vi "VCS Set Quick Stop State.vi"(8 "error in (no error)":errorcluster, 11 "axis in":cluster{"keyHandle":u32, "nodeId":u16}={"keyHandle"=0, "nodeId"=1}) -> (0 "error out":errorcluster, 3 "axis out":cluster{"keyHandle":u32, "nodeId":u16}={"keyHandle"=0, "nodeId"=1})   [LabVIEW 2019]
doc: "<B>VCS Set Quick Stop State</B> the device changes to quick stop state."
uses:
  Resources/EposCmd.dll
  Resources/EposCmd64.dll
panel:
  in  "pErrorCode":u32
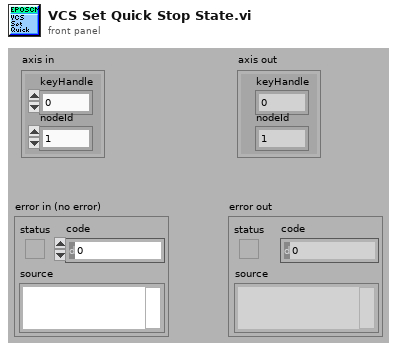
[diagram p1: front panel]
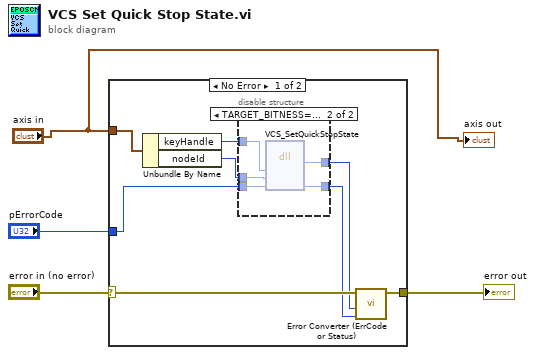
[diagram p0: block diagram]
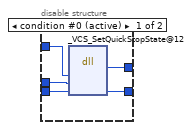
[diagram p2: hidden frame]
diagram:
  n1 = case shown="No Error" "error in (no error)" {
    selector: "error in (no error)" -> [w11 w23]
    tunnel: [w10 w23] -> w3
    tunnel: "pErrorCode" -> [w12 _]
    tunnel: "axis in" -> [w8 _]
    frame No Error {
      n2 = Unbundle By Name(w8) -> ("keyHandle"=w7:u32, "nodeId"=w6:u16)
      n3 = disable-structure shown="TARGET_BITNESS==64" {
        disable-tunnel: w12 -> [w17 w22]
        disable-tunnel: [w16 w21] -> w9
        disable-tunnel: w7 -> [w15 w20]
        disable-tunnel: w6 -> [w14 w19]
        disable-tunnel: [w13 w18] -> w5
        frame condition #0 (active) {
          n4 = dll-call lib="C:/Projeto em LabVIEW/EPOS-LabVIEW-Instrument-Driver-En/LabVIEW/maxon EPOS/Resources/EposCmd.*" fn="_VCS_SetQuickStopState@12"("KeyHandle"=w15, "NodeId"=w14, "pErrorCode"=w17) -> (w13:i32, "pErrorCode"=w16:u32)  [unwired: 5 in, 2 out]
        }
        frame condition #1 {
          n5 = dll-call lib="C:/setup/Resources/EposCmd64.*" fn="VCS_SetQuickStopState" ("EposCmd.dll:_VCS_SetQuickStopState@12")("KeyHandle"=w20, "NodeId"=w19, "pErrorCode"=w22) -> ("Rückgabetyp"=w18:i32, "pErrorCode"=w21:u32)  [unwired: 5 in, 2 out]
        }
      }
      n6 = call "Error Converter (ErrCode or Status).vi"("error code"=w9, "return type"=w5, "error in (no error)"=w11) -> ("error out"=w10:errorcluster)  [unwired: 7 in]
    }
    frame Error {
    }
  }
  "error out" <- w3
  "axis out" <- "axis in"
